vi "PSUN8731A-CTRLv3.vi"() -> ()   [LabVIEW 2017]
uses:
  <vilib>/Analysis/6fits.llb/Curve Fitting Criteria.ctl
  Controller subVIs/CurrentPSUSettings.vi
  Keysight N8731A conversion/Keysight N8900 Series.lvlib
  <vilib>/Analysis/NI_AALPro.lvlib
panel:
  out "Tr [s]":dbl
  in  "Quench Protection":bool
  out "Status message":string
  out "TimeData":dbl[](array[numeric])
  out "VoltData":dbl[](array[numeric])
  out "CurrData":dbl[](array[numeric])
  out "StartTime":dbl
  out "I(t)":cluster{dbl[], dbl[]}(graph)
  out "V(t)":cluster{dbl[], dbl[]}(graph)
  in  "Sweep Controller":enum32{"Sweep Mode", "Free Control Mode"}(tab)=enum."Free Control Mode"
  in  "Maximum Voltage [V]":dbl min=0.0 max=8.0 step=0.001
  in  "Maximum Current [A]":dbl min=0.0 max=400.0 step=0.1
  in  "Coil Voltage Limit [V]":dbl=0.005 min=0.0 step=0.001
  in  "Initial Voltage [V]":dbl min=0.0 max=8.0 step=0.001
  in  "Initial meas delay [ms]":u32=500 step=10
  in  "Tr meas time [s]":dbl=60.0 min=0.0
  out "Voltage offset [V]":dbl
  in  "Time between data points (ms)":i32=500 min=0
  out "Immediate Voltage (V)":dbl
  out "Immediate Current (A)":dbl
  in  "Voltage Set [V]":dbl min=0.0 max=8.0 step=0.001
  in  "Current Set [A]":dbl min=0.0 max=400.0 step=0.1
  in  "Voltmeter channel (6)":i32=6
  in  "End Program":bool
  in  "Stop Sweep":bool
  out "Voltmeter error message":errorcluster
  in  "Voltmeter Range (V)":dbl caption="0 for Auto range"
  in  "Voltmeter Address (16)":i16=16
  out "PSU error message":errorcluster
  in  "Start Sweep":bool
  in  "Sweepback":bool=TRUE
  in  "Power Output":bool
  in  "OC protection":bool
  in  "OV Value (10V)":dbl=10.0 min=0.5 max=10.0
  out "I(V) Graph":cluster{dbl[], dbl[]}(graph)
  in  "VISA resource name":refnum<visa-resource-name>="N8731APSU"
  in  "Filename":string caption="Leave empty to discard data.\nDon't touch during measurement"
  in  "PSU\nVoltage":bool=TRUE caption="Keithley\nVoltage"
  in  "OV protection":bool=TRUE
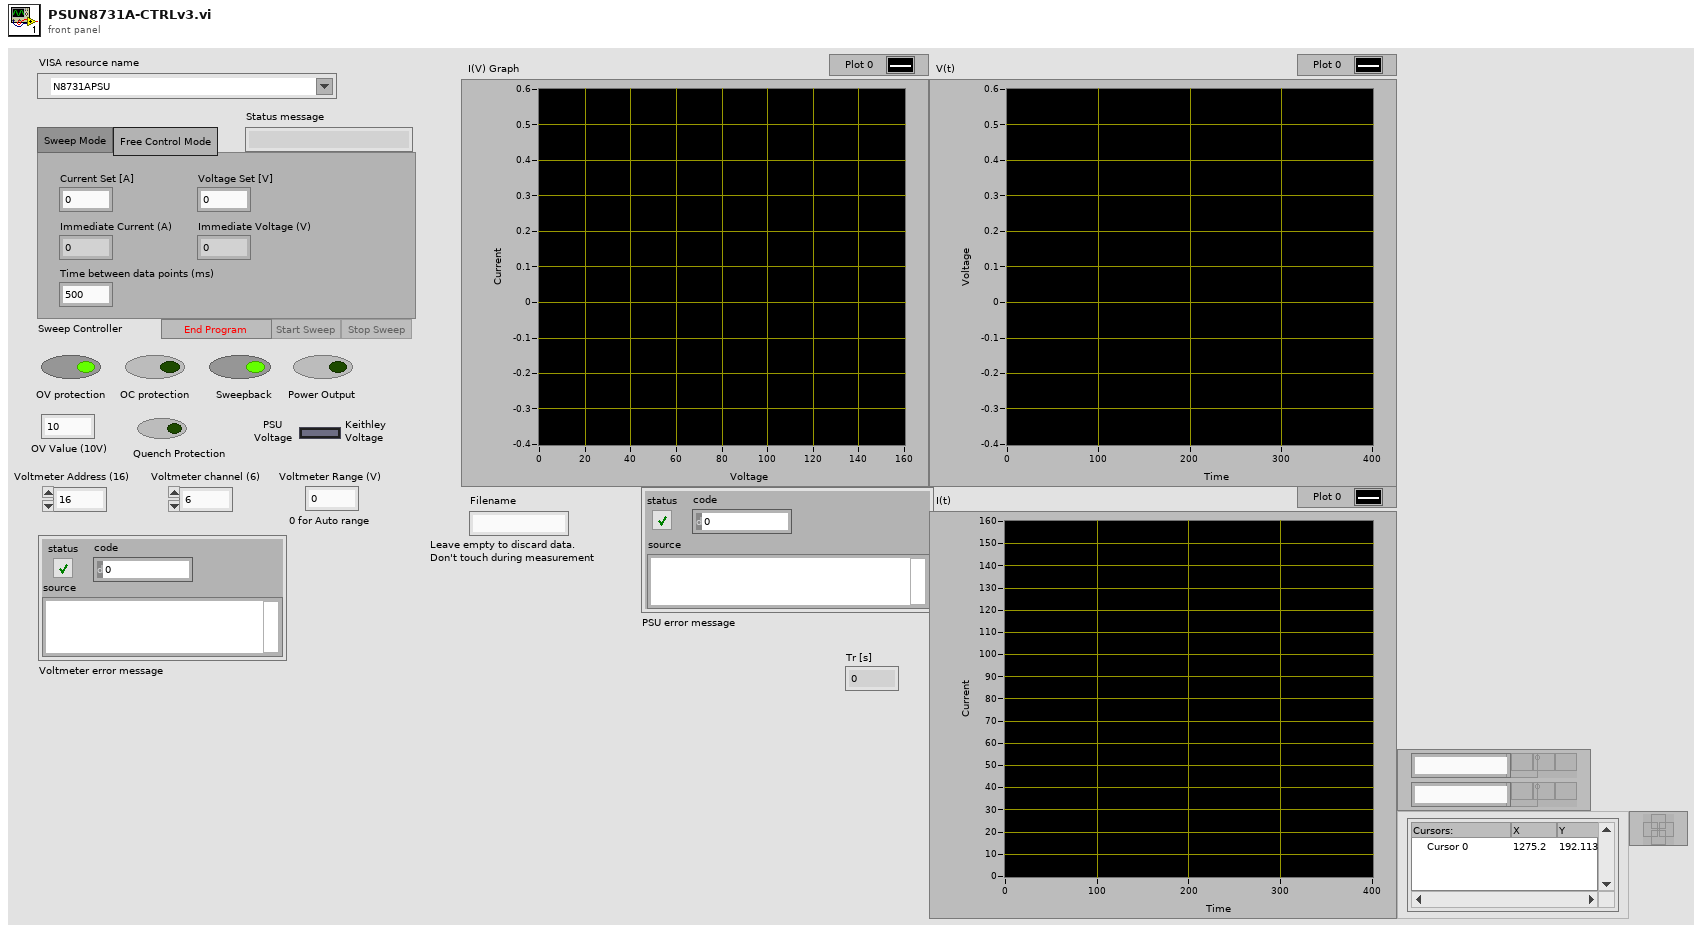
[diagram p1: front panel]
types:
  T1 = enum8{"Enabled", "Disabled", "Disabled and Grayed Out"}
  T2 = cluster{"amp min":dbl, "amp max":dbl, "damping min":dbl, "damping max":dbl, "offset min":dbl, "offset max":dbl}
  T3 = cluster{"Sweep Controller":enum32{"Sweep Mode", "Free Control Mode"}, "   PSU\nVoltage":bool}
  T4 = typedef "NI_AALPro.lvlib/Curve Fitting Criteria.ctl" = u16
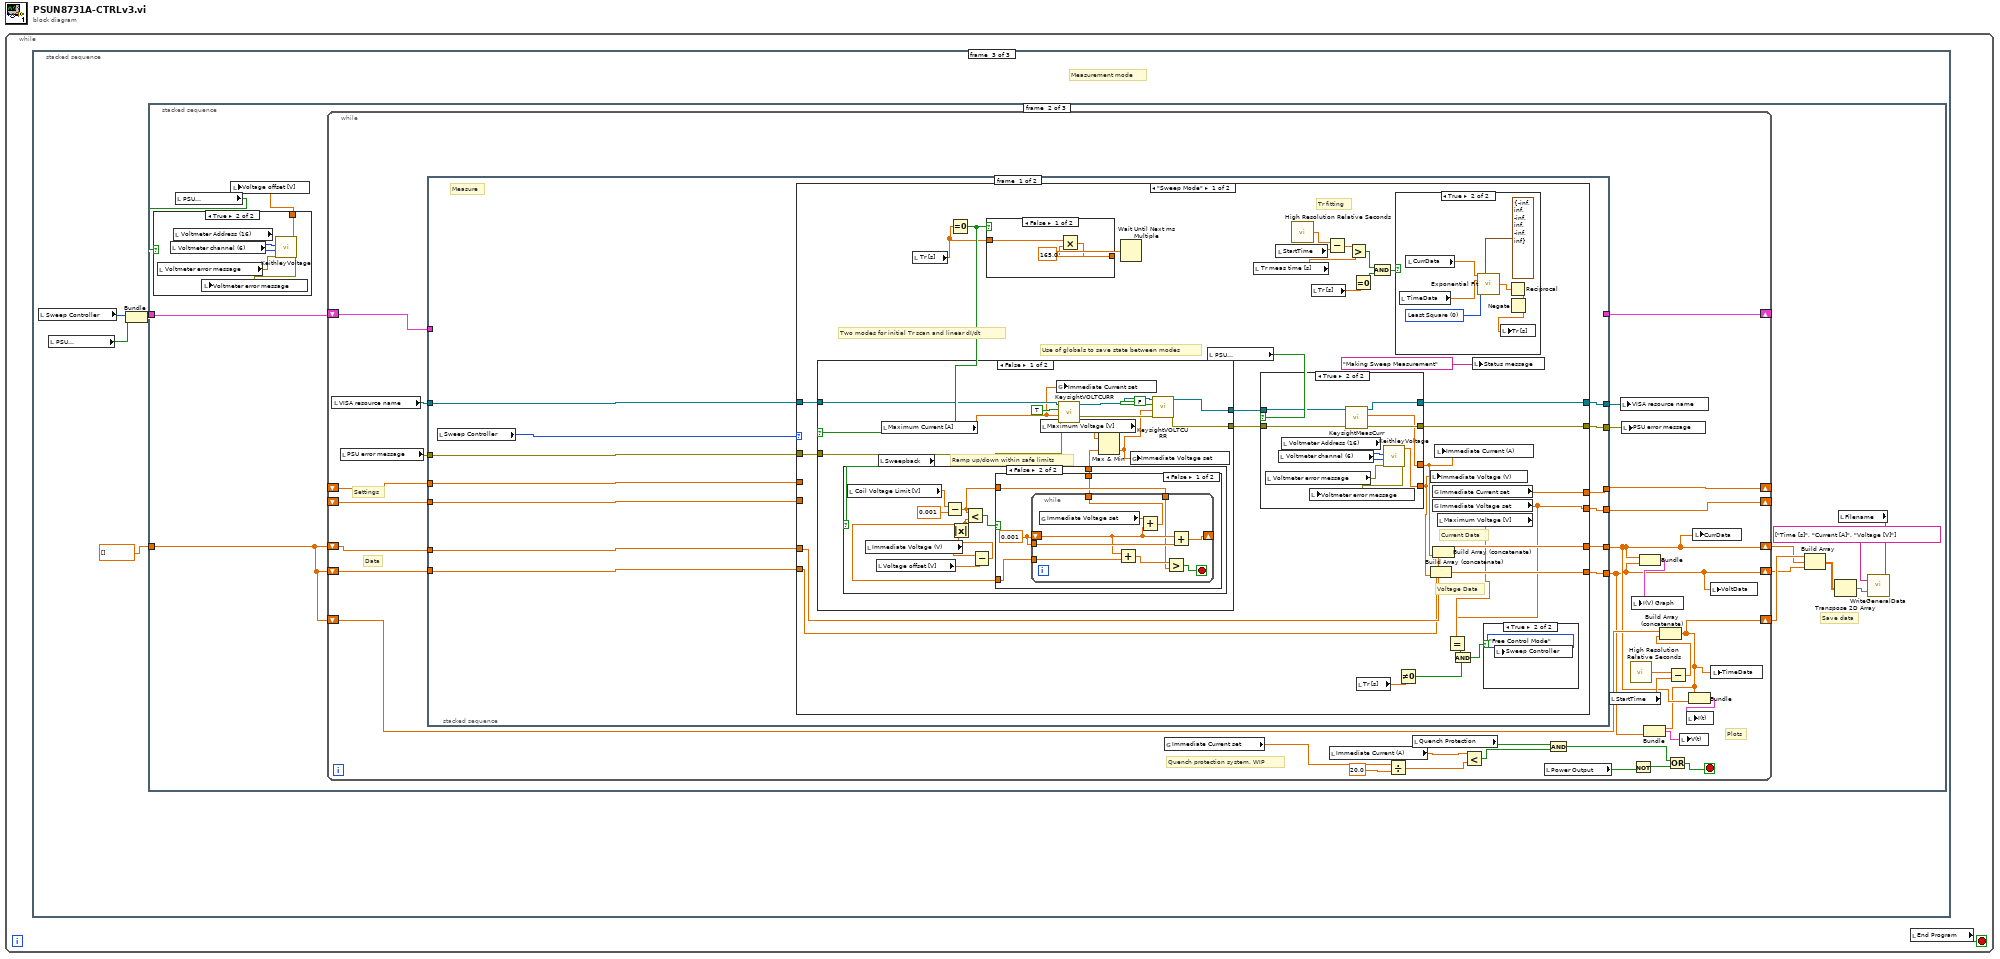
[diagram p0: block diagram]
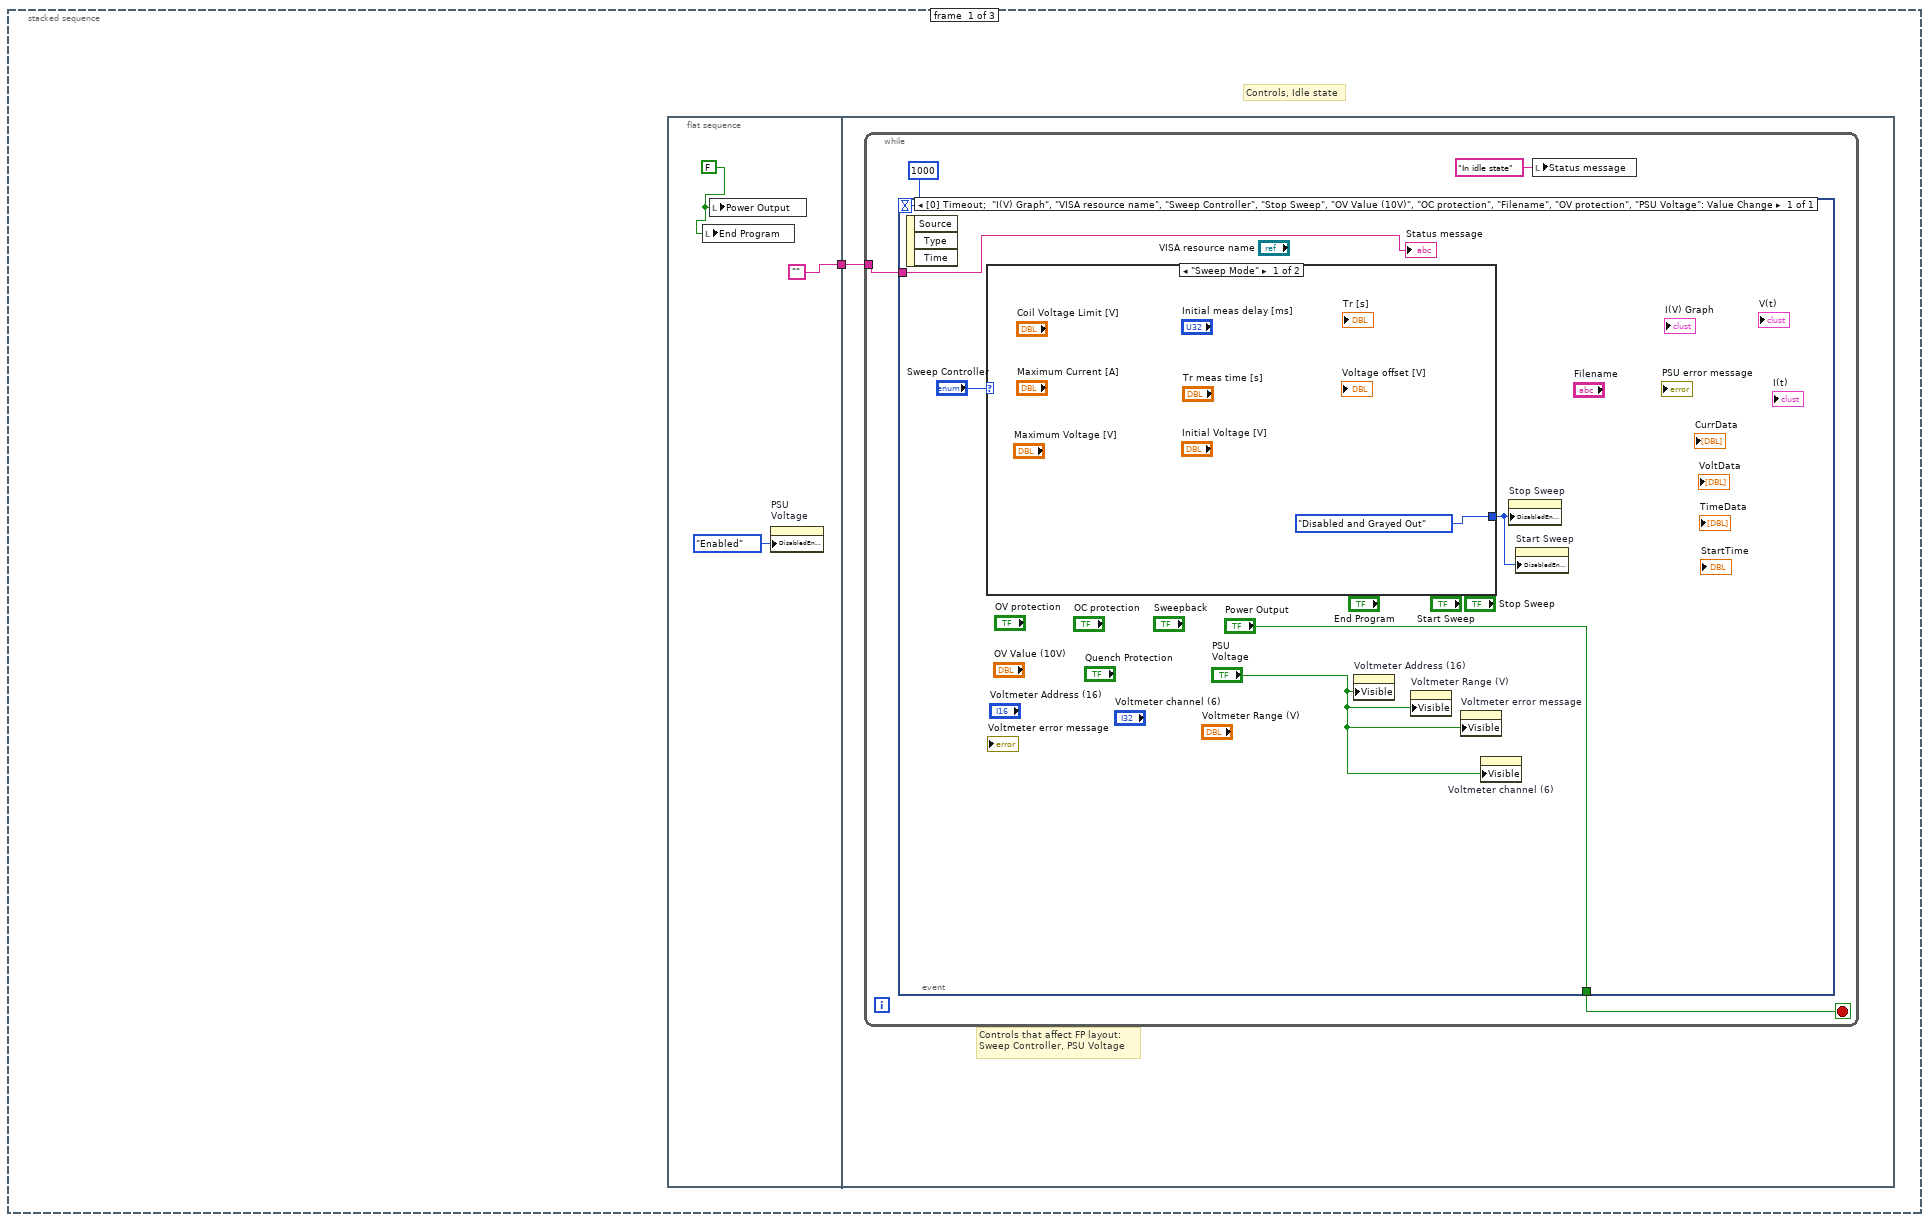
[diagram p2: hidden frame]
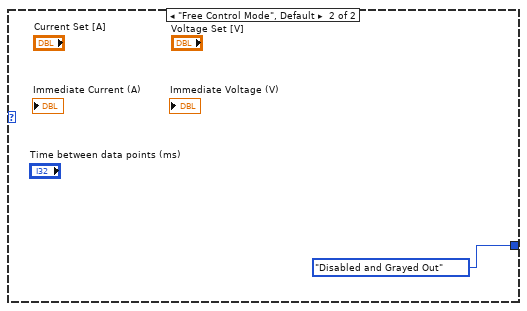
[diagram p3: hidden frame]
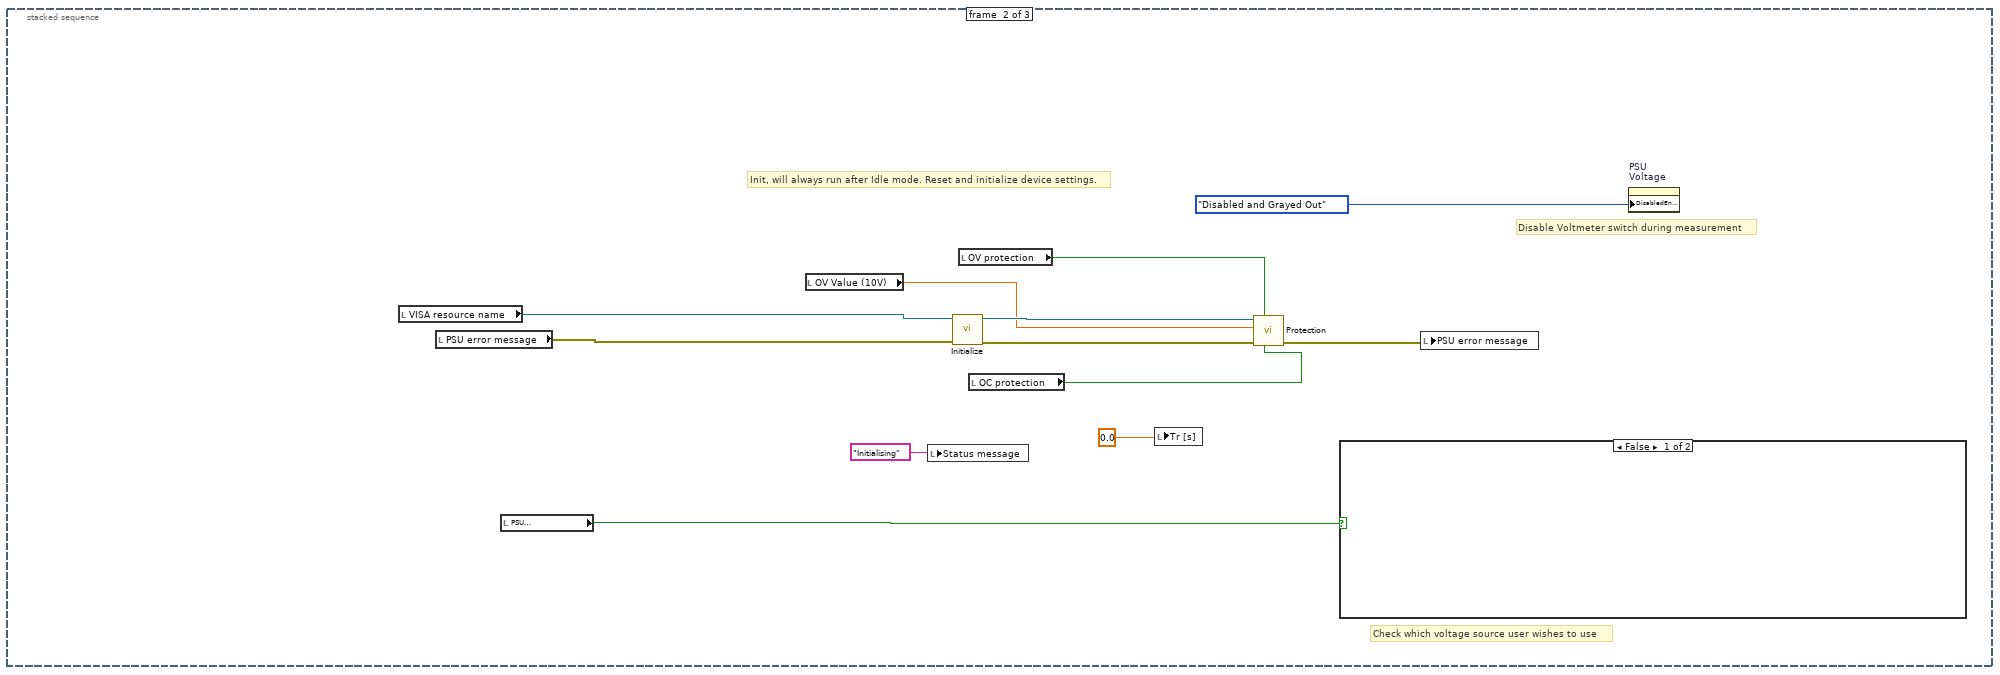
[diagram p4: hidden frame]
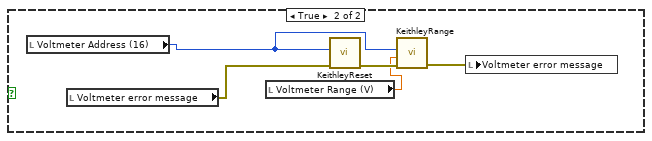
[diagram p5: hidden frame]
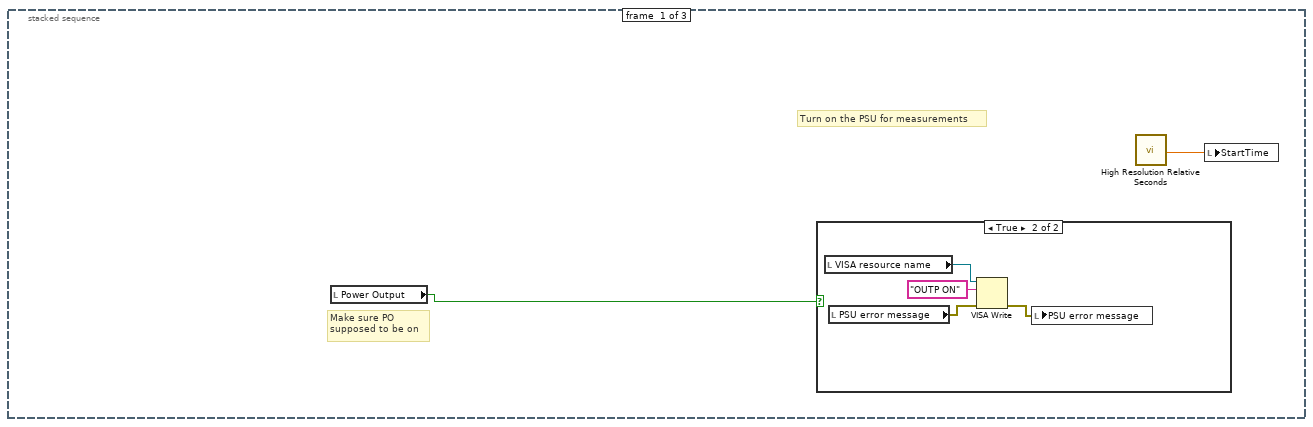
[diagram p6: hidden frame]
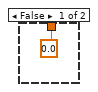
[diagram p8: hidden frame]
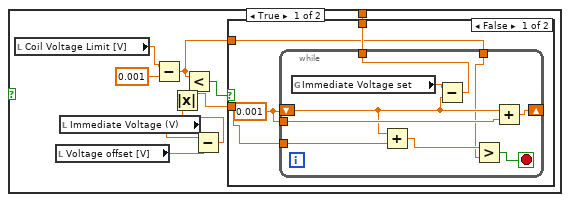
[diagram p10: hidden frame]
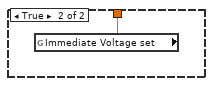
[diagram p11: hidden frame]
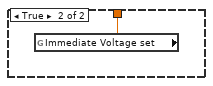
[diagram p12: hidden frame]
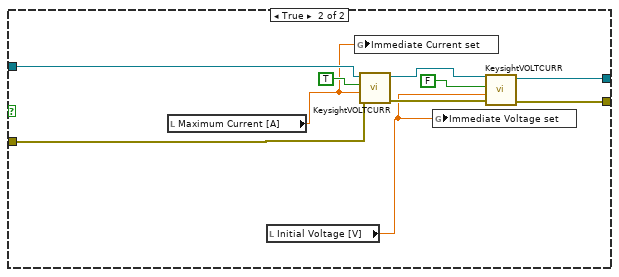
[diagram p13: hidden frame]
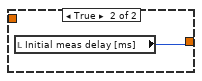
[diagram p15: hidden frame]
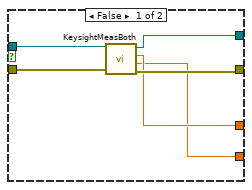
[diagram p16: hidden frame]
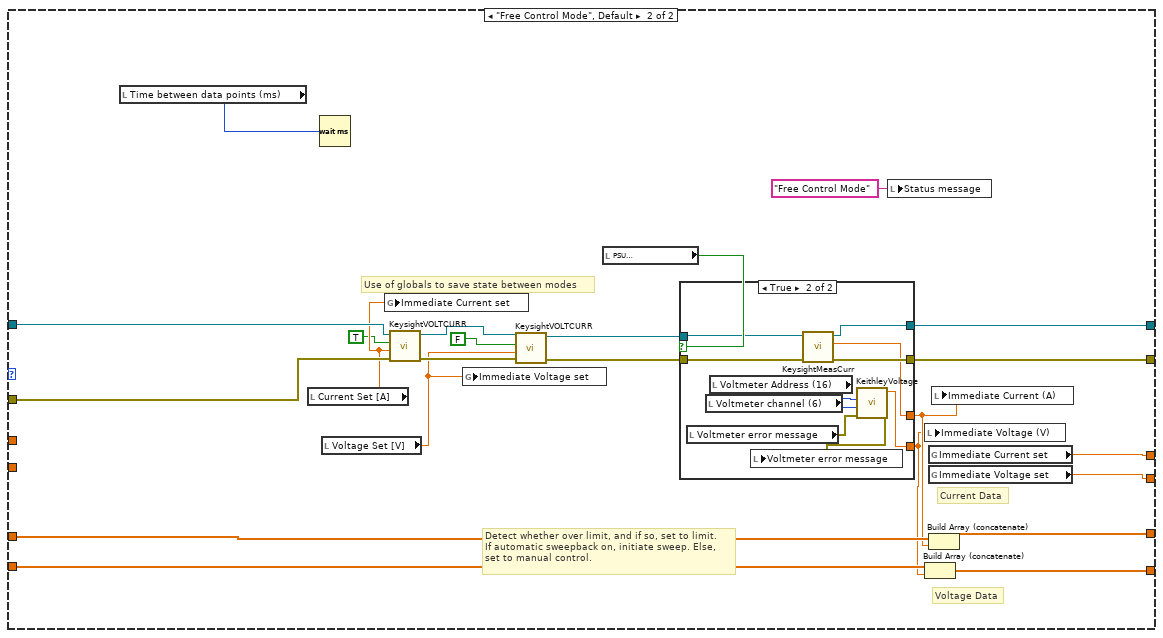
[diagram p17: hidden frame]
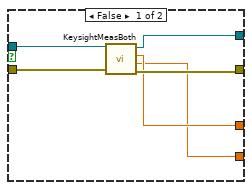
[diagram p18: hidden frame]
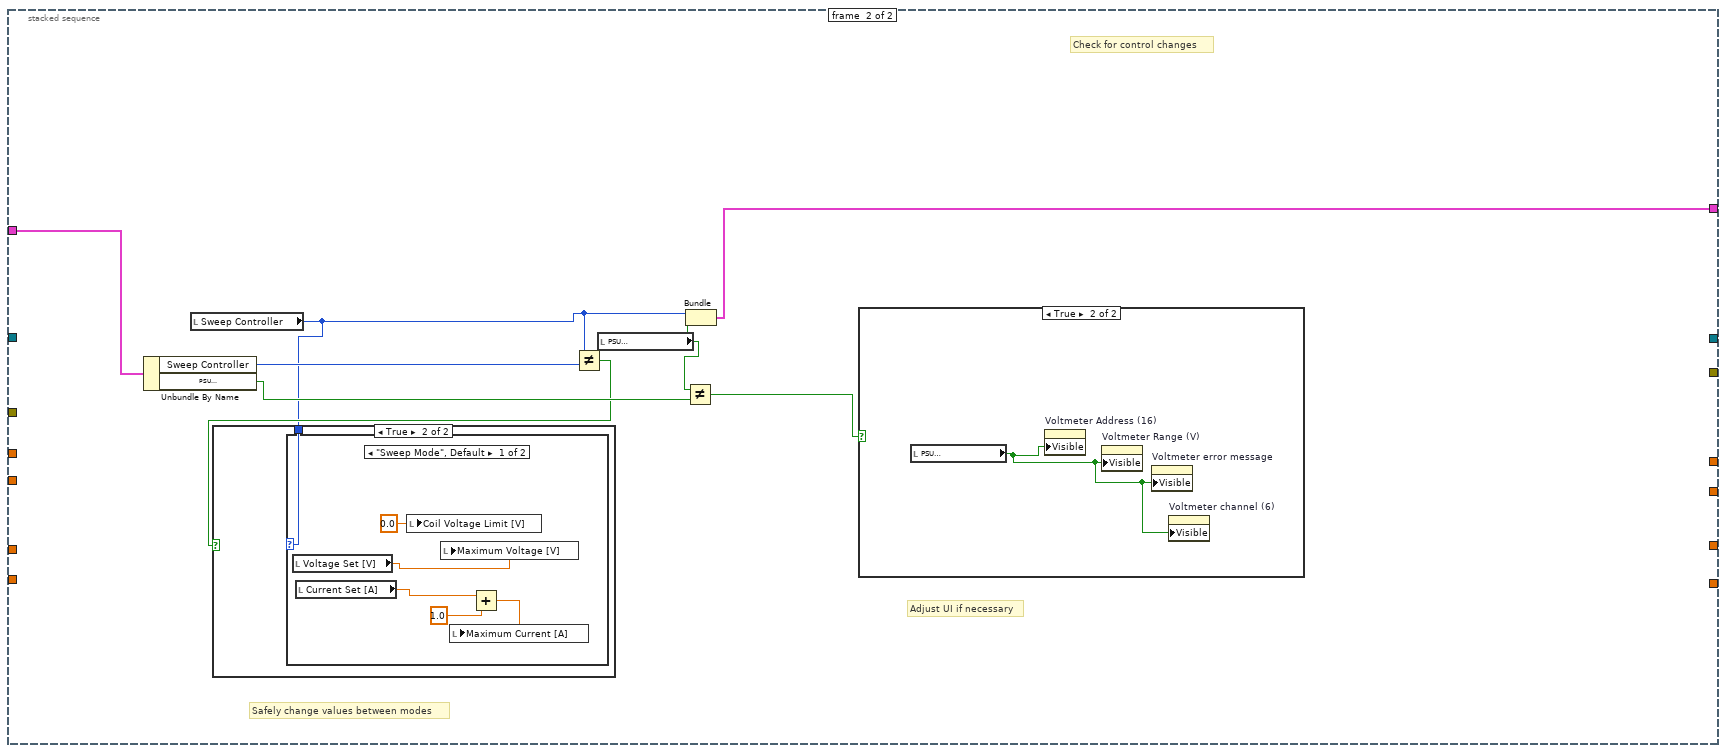
[diagram p19: hidden frame]
diagram:
  n1 = while {
    stop <- w1 stop-if-true
    n2 = stacked-sequence {
      frame #0 {
        # "Controls, Idle state"
        n3 = flat-sequence {
          tunnel: ["" ("Status message")] -> w2
          tunnel: w2 -> [w6]
          frame #0 {
            w3 = FALSE ("Sweeping Back")
            n4 = local write "End Program"(w3) -> ()
            n5 = local write "Power Output"(w3) -> ()
            n6 = property on="PSU\nVoltage" class="Bool (strict)"("DisabledEnum"=T1."Enabled" ("Disabled")) -> ()  [unwired: 2 in, 2 out]
          }
          frame #1 {
            # "Controls that affect FP layout:\nSweep Controller, PSU Voltage"
            n7 = while {
              tunnel: w6 -> [w8]
              stop <- w10 stop-if-true
              n8 = event shown="[0] Timeout;  \"I(V) Graph\", \"VISA resource name\", \"Sweep Controller\", \"Stop Sweep\", \"OV Value (10V)\", \"OC protection\", \"Filename\", \"OV protection\", \"PSU Voltage\": Value Change" {
                selector: _ -> [_]
                dyn-events: _ -> [_]
                timeout: 1000 -> [_]
                tunnel: ["Power Output"] -> w10
                tunnel: w8 -> [w11]
                event Timeout; "I(V) Graph", "VISA resource name", "Sweep Controller", "Stop Sweep", "OV Value (10V)", "OC protection", "Filename", "OV protection", "PSU\nVoltage": Value Change {
                  n9 = event-data() -> ()  [unwired: 1 in, 3 out]
                  n10 = case shown="\"Sweep Mode\"" "Sweep Controller" {
                    tunnel: [T1."Disabled and Grayed Out" ("Disabled") T1."Disabled and Grayed Out" ("Disabled")] -> w13
                    frame "Sweep Mode" {
                    }
                    frame "Free Control Mode", Default {
                    }
                  }
                  n11 = property on="Voltmeter Address (16)" class="DigNum (strict)"("Visible"="PSU\nVoltage") -> ()  [unwired: 2 in, 2 out]
                  n12 = property on="Voltmeter Range (V)" class="DigNum (strict)"("Visible"="PSU\nVoltage") -> ()  [unwired: 2 in, 2 out]
                  n13 = property on="Voltmeter error message" class="Clust (strict)"("Visible"="PSU\nVoltage") -> ()  [unwired: 2 in, 2 out]
                  n14 = property on="Voltmeter channel (6)" class="DigNum (strict)"("Visible"="PSU\nVoltage") -> ()  [unwired: 2 in, 2 out]
                  n15 = property on="Stop Sweep" class="Bool"("DisabledEnum"=w13) -> ()  [unwired: 2 in, 2 out]
                  n16 = property on="Start Sweep" class="Bool"("DisabledEnum"=w13) -> ()  [unwired: 2 in, 2 out]
                  "Status message" <- w11
                }
              }
              n17 = local write "Status message"("In idle state" ("Status message")) -> ()
            }
          }
        }
      }
      frame #1 {
        # "Check which voltage source user wishes to use"
        # "Disable Voltmeter switch during measurement"
        # "Init, will always run after Idle mode. Reset and initialize device settings."
        n18 = local read "VISA resource name"() -> (w27:refnum<visa-resource-name>)
        n19 = local read "PSU error message"() -> (w22:errorcluster)
        n20 = local read "PSU\nVoltage"() -> (w21:bool)
        n21 = local read "OV Value (10V)"() -> (w26:dbl)
        n22 = local write "Status message"("Initialising" ("Status message")) -> ()
        n23 = call "Initialize.vi"("error in (no error)"=w22, "VISA resource name"=w27) -> ("error out"=w28:errorcluster, "VISA resource name out"=w29:refnum<visa-resource-name>)  [unwired: 8 in]
        n24 = local read "OV protection"() -> (w24:bool)
        n25 = local read "OC protection"() -> (w25:bool)
        n26 = local write "Tr [s]"(0.0 ("Tr")) -> ()
        n27 = call "Protection.vi"("OC protection"=w25, "OV protection"=w24, "error in (no error)"=w28, "OV Value (10V)"=w26, "VISA resource name"=w29) -> ("error out"=w23:errorcluster)  [unwired: 5 in, 1 out]
        n28 = case shown="False" w21 {
          frame False {
          }
          frame True {
            n29 = local read "Voltmeter Address (16)"() -> (w30:i16)
            n30 = local read "Voltmeter error message"() -> (w32:errorcluster)
            n31 = local read "Voltmeter Range (V)"() -> (w31:dbl)
            n32 = call "KeithleyReset.vi"("error in"=w32, "address (16)"=w30) -> ("error out"=w33:errorcluster)  [unwired: 9 in]
            n33 = call "KeithleyRange.vi"("error in"=w33, "Range (V)/Auto(0)"=w31, "address (16)"=w30) -> ("error out"=w34:errorcluster)  [unwired: 8 in]
            n34 = local write "Voltmeter error message"(w34) -> ()
          }
        }
        n35 = local write "PSU error message"(w23) -> ()
        n36 = property on="PSU\nVoltage" class="Bool (strict)"("DisabledEnum"=T1."Disabled and Grayed Out" ("Disabled")) -> ()  [unwired: 2 in, 2 out]
      }
      frame #2 {
        # "Measurement mode"
        n37 = local read "Sweep Controller"() -> (w38:enum32{"Sweep Mode", "Free Control Mode"})
        n38 = local read "PSU\nVoltage"() -> (w37:bool)
        n39 = Bundle("Sweep Controller"=w38, "PSU\nVoltage"=w37) -> (w36:T3)  [unwired: 1 in]
        n40 = stacked-sequence {
          tunnel: w36 -> [_ w55 _]
          tunnel: dbl[] [] -> [_ w54 _]
          frame #0 {
            # "Make sure PO\nsupposed to be on"
            # "Turn on the PSU for measurements"
            n41 = local read "Power Output"() -> (w40:bool)
            n42 = case shown="True" w40 {
              frame False {
              }
              frame True {
                n43 = local read "VISA resource name"() -> (w43:refnum<visa-resource-name>)
                n44 = local read "PSU error message"() -> (w42:errorcluster)
                n45 = VISA Write(VISA resource name=w43, write buffer="OUTP ON", error in (no error)=w42) -> (error out=w41:errorcluster)  [unwired: 2 out]
                n46 = local write "PSU error message"(w41) -> ()
              }
            }
            n47 = call <vilib>:"High Resolution Relative Seconds.vi"() -> ("relative seconds"=w39:dbl)
            n48 = local write "StartTime"(w39) -> ()
          }
          frame #1 {
            # "Save data"
            n49 = local read "PSU\nVoltage"() -> (w53:bool)
            n50 = case shown="True" w53 {
              tunnel: [0.0 ("Voltage") w57] -> w52
              frame False {
              }
              frame True {
                n51 = local read "Voltmeter error message"() -> (w59:errorcluster)
                n52 = local read "Voltmeter channel (6)"() -> (w61:i32)
                n53 = local read "Voltmeter Address (16)"() -> (w60:i16)
                n54 = call "KeithleyVoltage.vi"("error in"=w59, "channel (6)"=w61, "address (16)"=w60) -> ("error out"=w58:errorcluster, "Voltage"=w57:dbl)  [unwired: 7 in]
                n55 = local write "Voltmeter error message"(w58) -> ()
              }
            }
            n56 = local write "Voltage offset [V]"(w52) -> ()
            n57 = while {
              shift-right: [w63] -> _
              shift-left: w55 -> [w93]
              shift-right: [w84] -> _
              shift-left: _ -> [w82]
              shift-right: [w85] -> _
              shift-left: _ -> [w90]
              shift-right: [w66] -> w48
              shift-left: w54 -> [w87]
              shift-right: [w65] -> w47
              shift-left: w54 -> [w86]
              shift-right: [w64] -> w49
              shift-left: w54 -> [w80]
              stop <- w67 stop-if-true
              # "Plots"
              # "Quench protection system, WIP"
              # "Data"
              # "Settings"
              n58 = local read "VISA resource name"() -> (w92:refnum<visa-resource-name>)
              n59 = local read "PSU error message"() -> (w91:errorcluster)
              n60 = stacked-sequence {
                tunnel: w93 -> [_ w281]
                tunnel: w92 -> [w105 _]
                tunnel: w91 -> [w104 _]
                tunnel: w90 -> [w103 _]
                tunnel: [w102 _] -> w89
                tunnel: [w101 _] -> w88
                tunnel: w87 -> [w100 _]
                tunnel: [w99 _] -> w66
                tunnel: w86 -> [w98 _]
                tunnel: [w97 _] -> w65
                tunnel: [w96 _] -> w85
                tunnel: [w95 _] -> w84
                tunnel: w82 -> [w94 _]
                tunnel: [_ w277] -> w63
                frame #0 {
                  # "Measure"
                  n61 = local read "Sweep Controller"() -> (w106:enum32{"Sweep Mode", "Free Control Mode"})
                  n62 = case shown="\"Sweep Mode\"" w106 {
                    tunnel: w105 -> [w138 w258]
                    tunnel: w104 -> [w137 w257]
                    tunnel: w103 -> [_ _]
                    tunnel: [w136 w256] -> w102
                    tunnel: [w135 w255] -> w101
                    tunnel: w100 -> [w134 w254]
                    tunnel: [w133 w253] -> w99
                    tunnel: w98 -> [w116 w252]
                    tunnel: [w132 w251] -> w97
                    tunnel: [w126 w239] -> w96
                    tunnel: [w111 w238] -> w95
                    tunnel: w94 -> [_ _]
                    frame "Sweep Mode" {
                      # "Tr fitting"
                      # "Two modes for initial Tr scan and linear dI/dt"
                      # "Use of globals to save state between modes"
                      # "Voltage Data"
                      # "Current Data"
                      n63 = local read "Tr [s]"() -> (w115:dbl)
                      n64 = Equal To 0?(x=w115) -> (x = 0?=w117:bool)
                      n65 = case shown="False" w117 {
                        tunnel: w138 -> [w152 w208]
                        tunnel: w137 -> [w151 w207]
                        tunnel: [w146 w202] -> w130
                        tunnel: [w145 w201] -> w129
                        frame False {
                          # "Ramp up/down within safe limits"
                          n66 = local read "Sweepback"() -> (w143:bool)
                          n67 = case shown="False" w143 {
                            tunnel: [w161 w184] -> w141
                            frame True {
                              n68 = local read "Coil Voltage Limit [V]"() -> (w156:dbl)
                              n69 = local read "Voltage offset [V]"() -> (w159:dbl)
                              n70 = local read "Immediate Voltage (V)"() -> (w160:dbl)
                              n71 = Subtract(x=w156, y=0.001) -> (x-y=w154:dbl)
                              n72 = Subtract(x=w160, y=w159) -> (x-y=w155:dbl)
                              n73 = Absolute Value(x=w155) -> (abs(x)=w153:dbl)
                              n74 = Less?(x=w154, y=w153) -> (x < y?=w158:bool)
                              n75 = case shown="False" w158 {
                                tunnel: [w164 w175] -> w161
                                tunnel: w154 -> [w163 _]
                                tunnel: w153 -> [w162 _]
                                frame False {
                                w165 = 0.001 ("y")
                                n76 = while {
                                shift-right: [w173] -> _
                                shift-left: w165 -> [w168]
                                tunnel: w165 -> [w172]
                                tunnel: [w171] -> w164
                                tunnel: w163 -> [w166]
                                tunnel: w162 -> [w169]
                                stop <- w174 stop-if-true
                                n77 = global read "CurrentPSUSettings.vi" "Immediate Voltage set"() -> (w170:dbl)
                                n78 = Add(x=w168, y=w169) -> (x+y=w167:dbl)
                                n79 = Subtract(x=w170, y=w168) -> (x-y=w171:dbl)
                                n80 = Greater?(x=w167, y=w166) -> (0:w174:bool)
                                n81 = Add(x=w168, y=w172) -> (x+y=w173:dbl)
                                }
                                }
                                frame True {
                                n82 = global read "CurrentPSUSettings.vi" "Immediate Voltage set"() -> (w175:dbl)
                                }
                              }
                            }
                            frame False {
                              n83 = local read "Coil Voltage Limit [V]"() -> (w179:dbl)
                              n84 = local read "Immediate Voltage (V)"() -> (w183:dbl)
                              n85 = local read "Voltage offset [V]"() -> (w182:dbl)
                              n86 = Subtract(x=w179, y=0.001) -> (x-y=w177:dbl)
                              n87 = Subtract(x=w183, y=w182) -> (x-y=w178:dbl)
                              n88 = Absolute Value(x=w178) -> (abs(x)=w176:dbl)
                              n89 = Less?(x=w177, y=w176) -> (x < y?=w181:bool)
                              n90 = case shown="False" w181 {
                                tunnel: [w186 w198] -> w184
                                tunnel: w177 -> [w188 _]
                                tunnel: w176 -> [w185 _]
                                frame False {
                                w187 = 0.001 ("y")
                                n91 = while {
                                shift-right: [w196] -> _
                                shift-left: w187 -> [w192]
                                tunnel: w188 -> [w189]
                                tunnel: w187 -> [w195]
                                tunnel: [w194] -> w186
                                tunnel: w185 -> [w191]
                                stop <- w197 stop-if-true
                                n92 = global read "CurrentPSUSettings.vi" "Immediate Voltage set"() -> (w193:dbl)
                                n93 = Add(x=w192, y=w191) -> (x+y=w190:dbl)
                                n94 = Add(x=w193, y=w192) -> (x+y=w194:dbl)
                                n95 = Greater?(x=w190, y=w189) -> (0:w197:bool)
                                n96 = Add(x=w192, y=w195) -> (x+y=w196:dbl)
                                }
                                }
                                frame True {
                                n97 = global read "CurrentPSUSettings.vi" "Immediate Voltage set"() -> (w198:dbl)
                                }
                              }
                            }
                          }
                          n98 = local read "Maximum Current [A]"() -> (w144:dbl)
                          n99 = local read "Maximum Voltage [V]"() -> (w142:dbl)
                          n100 = global write "CurrentPSUSettings.vi" "Immediate Current set"(w144) -> ()
                          n101 = call "KeysightVOLTCURR.vi"("error in (no error)"=w151, "CURR/VOLT (A/V)"=w144, "CURR (1)/VOLT (0)"=TRUE, "VISA resource name"=w152) -> ("error out"=w147:errorcluster, "VISA resource name out"=w148:refnum<visa-resource-name>)  [unwired: 6 in]
                          n102 = Max & Min(x=w142, y=w141) -> (min(x,y)=w140:dbl)  [unwired: 1 out]
                          n103 = global write "CurrentPSUSettings.vi" "Immediate Voltage set"(w140) -> ()
                          n104 = call "KeysightVOLTCURR.vi"("error in (no error)"=w147, "CURR/VOLT (A/V)"=w140, "CURR (1)/VOLT (0)"=FALSE, "VISA resource name"=w148) -> ("error out"=w145:errorcluster, "VISA resource name out"=w146:refnum<visa-resource-name>)  [unwired: 6 in]
                        }
                        frame True {
                          n105 = local read "Maximum Current [A]"() -> (w200:dbl)
                          n106 = local read "Initial Voltage [V]"() -> (w199:dbl)
                          n107 = global write "CurrentPSUSettings.vi" "Immediate Current set"(w200) -> ()
                          n108 = call "KeysightVOLTCURR.vi"("error in (no error)"=w207, "CURR/VOLT (A/V)"=w200, "CURR (1)/VOLT (0)"=TRUE, "VISA resource name"=w208) -> ("error out"=w203:errorcluster, "VISA resource name out"=w204:refnum<visa-resource-name>)  [unwired: 6 in]
                          n109 = global write "CurrentPSUSettings.vi" "Immediate Voltage set"(w199) -> ()
                          n110 = call "KeysightVOLTCURR.vi"("error in (no error)"=w203, "CURR/VOLT (A/V)"=w199, "CURR (1)/VOLT (0)"=FALSE, "VISA resource name"=w204) -> ("error out"=w201:errorcluster, "VISA resource name out"=w202:refnum<visa-resource-name>)  [unwired: 6 in]
                        }
                      }
                      n111 = case shown="False" w117 {
                        tunnel: [w217 w219] -> w125
                        tunnel: w115 -> [w216 _]
                        frame False {
                          n112 = Multiply(x=w216, y=165.0 ("Tr")) -> (x*y=w217:dbl)
                        }
                        frame True {
                          n113 = local read "Initial meas delay [ms]"() -> (w219:u32)
                        }
                      }
                      n114 = Wait Until Next ms Multiple(millisecond multiple=w125) -> ()  [unwired: 1 out]
                      n115 = local read "PSU\nVoltage"() -> (w131:bool)
                      n116 = local read "Tr meas time [s]"() -> (w114:dbl)
                      n117 = case shown="True" w131 {
                        tunnel: w130 -> [w225 w235]
                        tunnel: w129 -> [w224 w234]
                        tunnel: [w223 w229] -> w136
                        tunnel: [w222 w228] -> w135
                        tunnel: [w221 w227] -> w128
                        tunnel: [w220 w226] -> w127
                        frame False {
                          n118 = call "KeysightMeasBoth.vi"("error in (no error)"=w224, "VISA resource name"=w225) -> ("error out"=w222:errorcluster, "VOLT"=w220:dbl, "CURR"=w221:dbl, "VISA resource name out"=w223:refnum<visa-resource-name>)  [unwired: 6 in]
                        }
                        frame True {
                          n119 = local read "Voltmeter error message"() -> (w231:errorcluster)
                          n120 = local read "Voltmeter channel (6)"() -> (w233:i32)
                          n121 = local read "Voltmeter Address (16)"() -> (w232:i16)
                          n122 = call "KeysightMeasCurr.vi"("error in (no error)"=w234, "VISA resource name"=w235) -> ("error out"=w228:errorcluster, "CURR"=w227:dbl, "VISA resource name out"=w229:refnum<visa-resource-name>)  [unwired: 7 in]
                          n123 = call "KeithleyVoltage.vi"("error in"=w231, "channel (6)"=w233, "address (16)"=w232) -> ("error out"=w230:errorcluster, "Voltage"=w226:dbl)  [unwired: 7 in]
                          n124 = local write "Voltmeter error message"(w230) -> ()
                        }
                      }
                      n125 = local read "StartTime"() -> (w123:dbl)
                      n126 = call <vilib>:"High Resolution Relative Seconds.vi"() -> ("relative seconds"=w124:dbl)
                      n127 = local read "Tr [s]"() -> (w120:dbl)
                      n128 = Subtract(x=w124, y=w123) -> (x-y=w122:dbl)
                      n129 = Greater?(x=w122, y=w114) -> (0:w118:bool)
                      n130 = Equal To 0?(x=w120) -> (x = 0?=w119:bool)
                      n131 = local read "Tr [s]"() -> (w110:dbl)
                      n132 = And(x=w118, y=w119) -> (x .and. y?=w121:bool)
                      n133 = case shown="True" w121 {
                        frame False {
                        }
                        frame True {
                          w213 = T4 0 items=["Least Square", "Least Absolute Residual", "Bisquare"] ("method")
                          n134 = local read "TimeData"() -> (w214:dbl[])
                          n135 = local read "CurrData"() -> (w215:dbl[])
                          n136 = call <vilib>:"Exponential Fit.vi"("Y"=w215, "X"=w214, "method"=w213, "parameter bounds"=T2 {"amp min"=-inf, "amp max"=inf, "damping min"=-inf, "damping max"=inf, "offset min"=-inf, "offset max"=inf}) -> ("damping"=w212:dbl)  [unwired: 6 in, 5 out]
                          n137 = Reciprocal(x=w212) -> (1/x=w210:dbl)
                          n138 = Negate(x=w210) -> (-x=w209:dbl)
                          n139 = local write "Tr [s]"(w209) -> ()
                        }
                      }
                      n140 = Not Equal To 0?(x=w110) -> (x != 0?=w108:bool)
                      n141 = local write "Immediate Voltage (V)"(w127) -> ()
                      n142 = Build Array (concatenate)(w116, w127) -> (w132:dbl[])
                      n143 = global read "CurrentPSUSettings.vi" "Immediate Current set"() -> (w126:dbl)
                      n144 = global read "CurrentPSUSettings.vi" "Immediate Voltage set"() -> (w111:dbl)
                      n145 = Build Array (concatenate)(w134, w128) -> (w133:dbl[])
                      n146 = local write "Immediate Current (A)"(w128) -> ()
                      n147 = local read "Maximum Voltage [V]"() -> (w112:dbl)
                      n148 = Equal?(x=w111, y=w112) -> (x = y?=w109:bool)
                      n149 = And(x=w109, y=w108) -> (x .and. y?=w107:bool)
                      n150 = local write "Status message"("Making Sweep Measurement" ("Status message")) -> ()
                      n151 = case shown="True" w107 {
                        frame False {
                        }
                        frame True {
                          n152 = local write "Sweep Controller"(enum32{"Sweep Mode", "Free Control Mode"}."Free Control Mode" ("Sweep Controller")) -> ()
                        }
                      }
                    }
                    frame "Free Control Mode", Default {
                      # "Use of globals to save state between modes"
                      # "Detect whether over limit, and if so, set to limit.\nIf automatic sweepback on, initiate sweep. Else,\nset to manual control."
                      # "Voltage Data"
                      # "Current Data"
                      n153 = local read "Time between data points (ms)"() -> (w237:i32)
                      n154 = local read "Current Set [A]"() -> (w250:dbl)
                      n155 = Wait (ms)(milliseconds to wait=w237) -> ()  [unwired: 1 out]
                      n156 = local read "Voltage Set [V]"() -> (w241:dbl)
                      n157 = global write "CurrentPSUSettings.vi" "Immediate Current set"(w250) -> ()
                      n158 = call "KeysightVOLTCURR.vi"("error in (no error)"=w257, "CURR/VOLT (A/V)"=w250, "CURR (1)/VOLT (0)"=TRUE, "VISA resource name"=w258) -> ("error out"=w246:errorcluster, "VISA resource name out"=w247:refnum<visa-resource-name>)  [unwired: 6 in]
                      n159 = global write "CurrentPSUSettings.vi" "Immediate Voltage set"(w241) -> ()
                      n160 = call "KeysightVOLTCURR.vi"("error in (no error)"=w246, "CURR/VOLT (A/V)"=w241, "CURR (1)/VOLT (0)"=FALSE, "VISA resource name"=w247) -> ("error out"=w243:errorcluster, "VISA resource name out"=w244:refnum<visa-resource-name>)  [unwired: 6 in]
                      n161 = local read "PSU\nVoltage"() -> (w245:bool)
                      n162 = case shown="True" w245 {
                        tunnel: w244 -> [w264 w274]
                        tunnel: w243 -> [w263 w273]
                        tunnel: [w262 w268] -> w256
                        tunnel: [w261 w267] -> w255
                        tunnel: [w260 w266] -> w242
                        tunnel: [w259 w265] -> w240
                        frame False {
                          n163 = call "KeysightMeasBoth.vi"("error in (no error)"=w263, "VISA resource name"=w264) -> ("error out"=w261:errorcluster, "VOLT"=w259:dbl, "CURR"=w260:dbl, "VISA resource name out"=w262:refnum<visa-resource-name>)  [unwired: 6 in]
                        }
                        frame True {
                          n164 = local read "Voltmeter error message"() -> (w270:errorcluster)
                          n165 = local read "Voltmeter channel (6)"() -> (w272:i32)
                          n166 = local read "Voltmeter Address (16)"() -> (w271:i16)
                          n167 = call "KeysightMeasCurr.vi"("error in (no error)"=w273, "VISA resource name"=w274) -> ("error out"=w267:errorcluster, "CURR"=w266:dbl, "VISA resource name out"=w268:refnum<visa-resource-name>)  [unwired: 7 in]
                          n168 = call "KeithleyVoltage.vi"("error in"=w270, "channel (6)"=w272, "address (16)"=w271) -> ("error out"=w269:errorcluster, "Voltage"=w265:dbl)  [unwired: 7 in]
                          n169 = local write "Voltmeter error message"(w269) -> ()
                        }
                      }
                      n170 = local write "Status message"("Free Control Mode" ("Status message")) -> ()
                      n171 = local write "Immediate Voltage (V)"(w240) -> ()
                      n172 = Build Array (concatenate)(w252, w240) -> (w251:dbl[])
                      n173 = global read "CurrentPSUSettings.vi" "Immediate Current set"() -> (w239:dbl)
                      n174 = global read "CurrentPSUSettings.vi" "Immediate Voltage set"() -> (w238:dbl)
                      n175 = Build Array (concatenate)(w254, w242) -> (w253:dbl[])
                      n176 = local write "Immediate Current (A)"(w242) -> ()
                    }
                  }
                }
                frame #1 {
                  # "Safely change values between modes"
                  # "Adjust UI if necessary"
                  # "Check for control changes"
                  n177 = Unbundle By Name(w281) -> ("Sweep Controller"=w282:enum32{"Sweep Mode", "Free Control Mode"}, "PSU\nVoltage"=w279:bool)
                  n178 = local read "Sweep Controller"() -> (w275:enum32{"Sweep Mode", "Free Control Mode"})
                  n179 = Not Equal?(x=w275, y=w282) -> (x != y?=w276:bool)
                  n180 = case shown="True" w276 {
                    tunnel: w275 -> [_ w283]
                    frame False {
                    }
                    frame True {
                      n181 = case shown="\"Sweep Mode\", Default" w283 {
                        frame "Sweep Mode", Default {
                          n182 = local read "Voltage Set [V]"() -> (w284:dbl)
                          n183 = local read "Current Set [A]"() -> (w285:dbl)
                          n184 = local write "Coil Voltage Limit [V]"(0.0 ("Coil Voltage Limit [V]")) -> ()
                          n185 = local write "Maximum Voltage [V]"(w284) -> ()
                          n186 = Add(x=w285, y=1.0) -> (x+y=w286:dbl)
                          n187 = local write "Maximum Current [A]"(w286) -> ()
                        }
                        frame "Free Control Mode" {
                          n188 = global read "CurrentPSUSettings.vi" "Immediate Current set"() -> (w291:dbl)
                          n189 = global read "CurrentPSUSettings.vi" "Immediate Voltage set"() -> (w292:dbl)
                          n190 = local read "Tr [s]"() -> (w290:dbl)
                          n191 = Not Equal To 0?(x=w290) -> (x != 0?=w289:bool)
                          n192 = case shown="True" w289 {
                            tunnel: w290 -> [_ w294]
                            frame False {
                            }
                            frame True {
                              n193 = Multiply(x=w294, y=1000.0) -> (x*y=w293:dbl)
                              n194 = local write "Time between data points (ms)"(w293) -> ()
                            }
                          }
                          n195 = local write "Current Set [A]"(w291) -> ()
                          n196 = local write "Voltage Set [V]"(w292) -> ()
                        }
                      }
                    }
                  }
                  n197 = local read "PSU\nVoltage"() -> (w280:bool)
                  n198 = Not Equal?(x=w280, y=w279) -> (x != y?=w278:bool)
                  n199 = Bundle("Sweep Controller"=w275, "PSU\nVoltage"=w280) -> (w277:T3)  [unwired: 1 in]
                  n200 = case shown="True" w278 {
                    frame False {
                    }
                    frame True {
                      n201 = local read "PSU\nVoltage"() -> (w296:bool)
                      n202 = property on="Voltmeter Address (16)" class="DigNum (strict)"("Visible"=w296) -> ()  [unwired: 2 in, 2 out]
                      n203 = property on="Voltmeter Range (V)" class="DigNum (strict)"("Visible"=w296) -> ()  [unwired: 2 in, 2 out]
                      n204 = property on="Voltmeter error message" class="Clust (strict)"("Visible"=w296) -> ()  [unwired: 2 in, 2 out]
                      n205 = property on="Voltmeter channel (6)" class="DigNum (strict)"("Visible"=w296) -> ()  [unwired: 2 in, 2 out]
                    }
                  }
                }
              }
              n206 = global read "CurrentPSUSettings.vi" "Immediate Current set"() -> (w72:dbl)
              n207 = local read "Immediate Current (A)"() -> (w73:dbl)
              n208 = Divide(x=w72, y=20.0) -> (x/y=w70:dbl)
              n209 = local read "Quench Protection"() -> (w62:bool)
              n210 = Less?(x=w73, y=w70) -> (x < y?=w74:bool)
              n211 = local read "Power Output"() -> (w81:bool)
              n212 = And(x=w62, y=w74) -> (x .and. y?=w68:bool)
              n213 = local read "StartTime"() -> (w78:dbl)
              n214 = local write "VISA resource name"(w89) -> ()
              n215 = local write "PSU error message"(w88) -> ()
              n216 = call <vilib>:"High Resolution Relative Seconds.vi"() -> ("relative seconds"=w79:dbl)
              n217 = Not(x=w81) -> (.not. x?=w69:bool)
              n218 = Bundle(w66, w65) -> (w83:cluster{dbl[], dbl[]})  [unwired: 1 in]
              n219 = local write "I(V) Graph"(w83) -> ()
              n220 = Or(x=w68, y=w69) -> (x .or. y?=w67:bool)
              n221 = Subtract(x=w79, y=w78) -> (x-y=w77:dbl)
              n222 = Build Array (concatenate)(w80, w77) -> (w64:dbl[])
              n223 = Bundle(w64, w65) -> (w76:cluster{dbl[], dbl[]})  [unwired: 1 in]
              n224 = local write "V(t)"(w76) -> ()
              n225 = Bundle(w64, w66) -> (w75:cluster{dbl[], dbl[]})  [unwired: 1 in]
              n226 = local write "I(t)"(w75) -> ()
              n227 = local write "CurrData"(w66) -> ()
              n228 = local write "VoltData"(w65) -> ()
              n229 = local write "TimeData"(w64) -> ()
            }
            n230 = Build Array(w49, w48, w47) -> (w45:dbl[][])
            n231 = Transpose 2D Array(2D array=w45) -> (transposed array=w46:dbl[][])
            n232 = local read "Filename"() -> (w51:string)
            n233 = call "WriteGeneralData.vi"("filename (discard if empty)"=w51, "Array"=w46, "Column name array"=string[] ["Time [s]", "Current [A]", "Voltage [V]"]) -> ()
          }
          frame #2 {
            # "Turn off PSU after measurements"
            n234 = local read "VISA resource name"() -> (w302:refnum<visa-resource-name>)
            n235 = local read "PSU error message"() -> (w301:errorcluster)
            n236 = VISA Write(VISA resource name=w302, write buffer="OUTP OFF", error in (no error)=w301) -> (VISA resource name out=w299:refnum<visa-resource-name>, error out=w298:errorcluster)  [unwired: 1 out]
            n237 = call "Close.vi"("error in (no error)"=w298, "VISA resource name"=w299) -> ("error out"=w297:errorcluster)  [unwired: 9 in]
            n238 = local write "PSU error message"(w297) -> ()
          }
        }
      }
    }
    n239 = local read "End Program"() -> (w1:bool)
  }
